vi "Configure Limit Test.vi"(4 "Limit Line Clip (T: Enable)":bool=TRUE, 6 "Limit Line Display (F: Disable)":bool, 7 "Limit Test (F: Disable)":bool, 8 "error in (no error)":errorcluster, 9 "Limit Fail Display (F: Disable)":bool, 10 "Channel (1)":i32=1, 11 "VISA resource name":refnum<visa-resource-name>) -> (0 "error out":errorcluster, 3 "VISA resource name out":refnum<visa-resource-name>)   [LabVIEW 2020, in "Agilent ENA Series.lvlib"]
doc: "Configures limit test parameters."
uses:
  <instrlib>/Agilent ENA Series/Agilent ENA Series.lvlib
panel:
  # "Enable\n\nDisable"
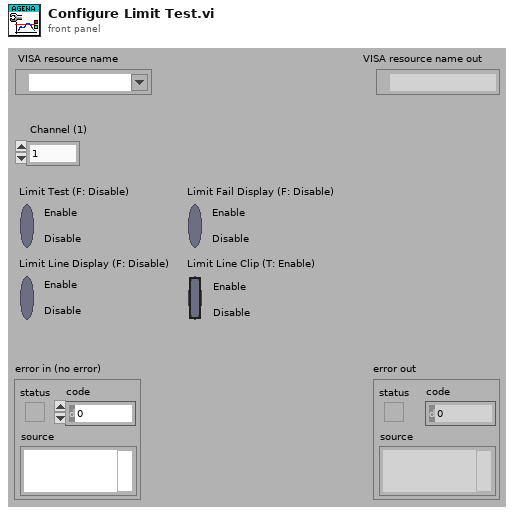
[diagram p1: front panel]
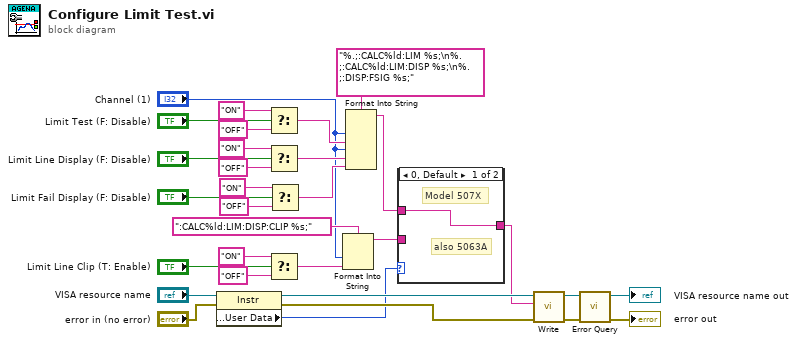
[diagram p0: block diagram]
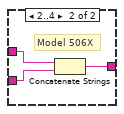
[diagram p2: hidden frame]
diagram:
  n1 = property class="Instr"(reference="VISA resource name", error in="error in (no error)") -> (reference out=w12:refnum<visa-resource-name>, error out=w11:errorcluster, "General Settings:User Data"=w4:u32)
  n2 = Select(t="ON", s="Limit Test (F: Disable)", f="OFF") -> (s? t:f=w24:string)
  n3 = Select(t="ON", s="Limit Line Display (F: Disable)", f="OFF") -> (s? t:f=w23:string)
  n4 = Select(t="ON", s="Limit Line Clip (T: Enable)", f="OFF") -> (s? t:f=w6:string)
  n5 = Select(t="ON", s="Limit Fail Display (F: Disable)", f="OFF") -> (s? t:f=w19:string)
  n6 = Format Into String(format string=":CALC%ld:LIM:DISP:CLIP %s;", "Channel (1)", w6) -> (resulting string=w3:string)  [unwired: 2 in, 1 out]
  n7 = Format Into String(format string="%.;:CALC%ld:LIM %s;\n%.;:CALC%ld:LIM:DISP %s;\n%.;:DISP:FSIG %s;", "Channel (1)", w24, "Channel (1)", w23, w19) -> (resulting string=w2:string)  [unwired: 2 in, 1 out]
  n8 = case shown="0, Default" w4 {
    tunnel: w3 -> [_ w34]
    tunnel: w2 -> [w32 w35]
    tunnel: [w32 w33] -> w1
    frame 0, Default {
      # "also 5063A"
      # "Model 507X"
    }
    frame 2..4 {
      # "Model 506X"
      n9 = Concatenate Strings(w35, w34) -> (w33:string)
    }
  }
  n10 = call <instrlib>:"Write.vi"("error in (no error)"=w11, "String ()"=w1, "VISA resource name"=w12) -> ("error out"=w17:errorcluster, "VISA resource name out"=w18:refnum<visa-resource-name>)  [unwired: 6 in, 1 out]
  n11 = call <instrlib>:"Error Query.vi"("error in (no error)"=w17, "VISA resource name"=w18) -> ("error out"=→"error out":errorcluster, "VISA resource name out"=→"VISA resource name out":refnum<visa-resource-name>)  [unwired: 6 in, 2 out]
